vi "listbox_set_values_and_recolor.vi"(4 "item_names":string[][](array[string]), 5 "uneditable_columns":string[](array[string]), 6 "front_panel_reference":refnum<vi>, 7 "column_names":string[](array[string]), 8 "error_in":errorcluster, 9 "Autosize? (T)":bool=TRUE, 10 "Recolor? (T)":bool=TRUE, 11 "multicolumn_listbox_reference_in":refnum<vi>) -> (0 "error_out":errorcluster, 3 "multicolumn_listbox_reference_out":refnum<vi>)   [LabVIEW 2020]
uses:
  <vilib>/Utility/miscctls.llb/LVRowAndColumnTypeDef.ctl
  <vilib>/Utility/miscctls.llb/LVRowAndColumnUnsignedTypeDef.ctl
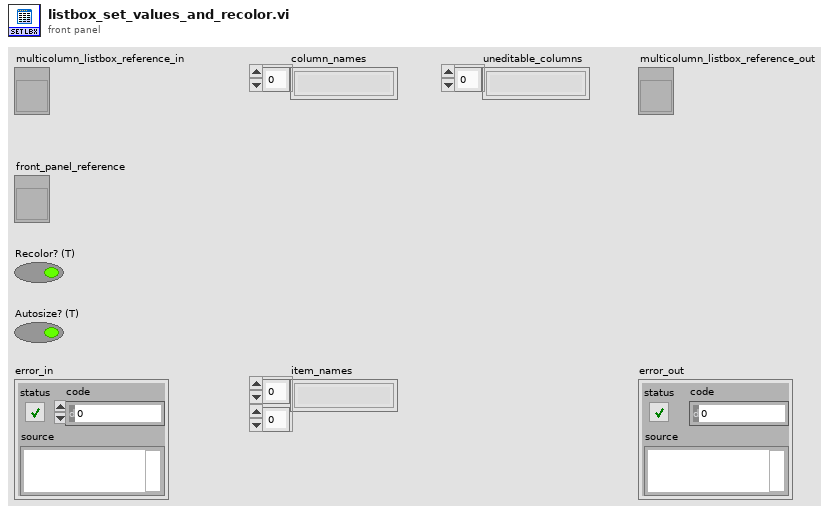
[diagram p1: front panel]
types:
  T1 = typedef "LVRowAndColumnUnsignedTypeDef.ctl" = cluster{"Row":u32, "Column":u32}
  T2 = typedef "LVRowAndColumnTypeDef.ctl" = cluster{"Row":i32, "Column":i32}
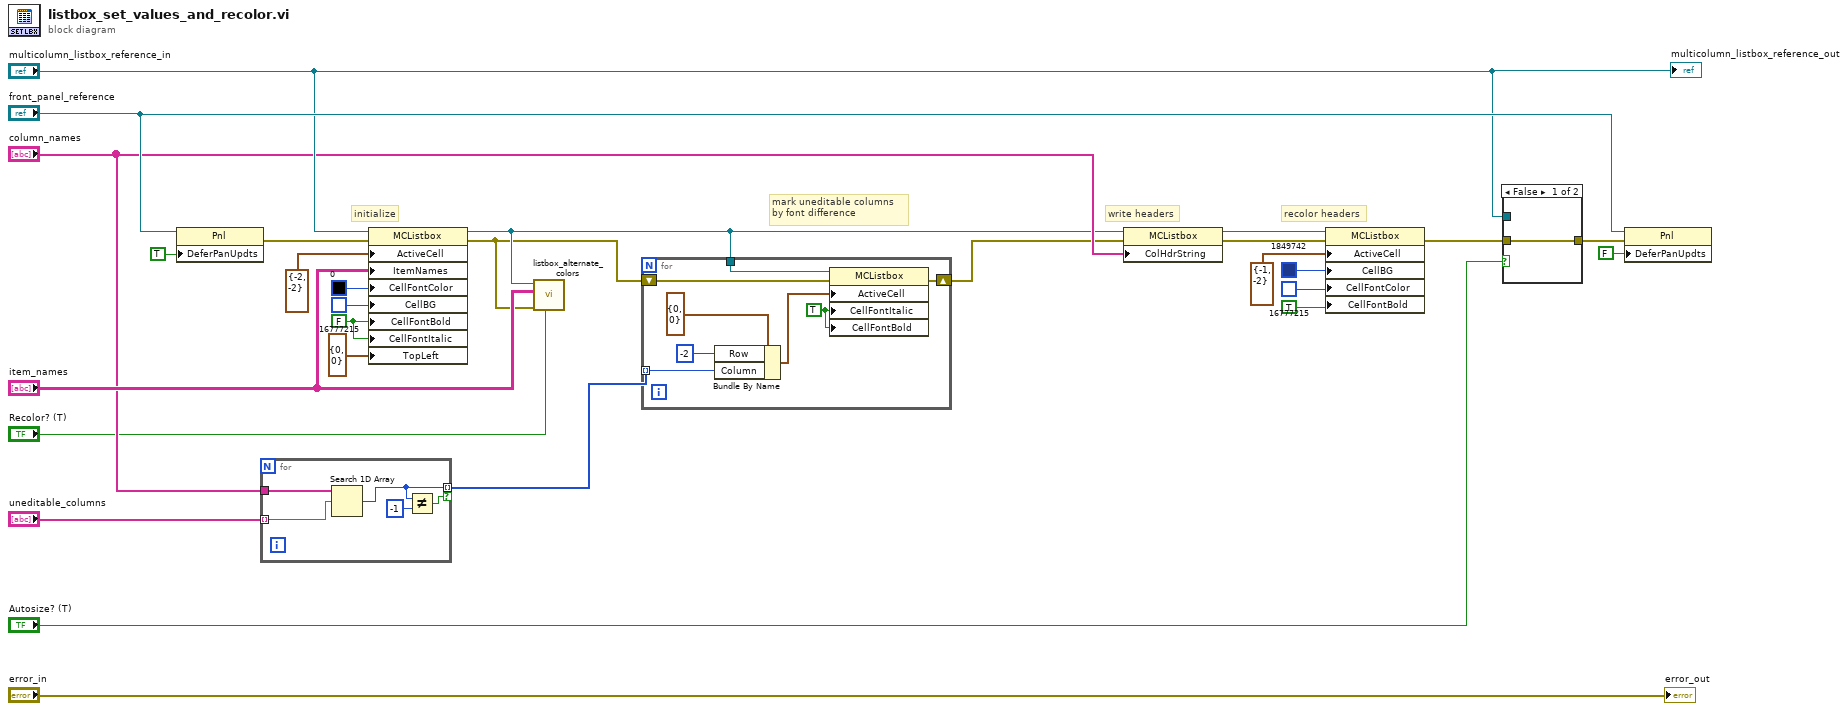
[diagram p0: block diagram]
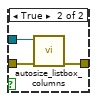
[diagram p2: hidden frame]
diagram:
  w6 = FALSE ("Active Cell:Cell Font:Bold")
  # "mark uneditable columns\nby font difference"
  # "recolor headers"
  # "write headers"
  # "initialize"
  n1 = property on="Property Node" class="Pnl"(reference="front_panel_reference", "DeferPanUpdts"=TRUE ("Defer Panel Updates")) -> (error out=w24:errorcluster)  [unwired: 1 in, 1 out]
  n2 = for {
    tunnel: "column_names" -> [w33]
    tunnel: "uneditable_columns" -> [w32] mode=indexing
    tunnel: [w30] -> w7 mode=indexing if=w31
    n3 = Search 1D Array(1D array=w33, element=w32) -> (index of element=w30:i32)  [unwired: 1 in]
    n4 = Not Equal?(x=w30, y=-1) -> (x != y?=w31:bool)
  }
  n5 = property on="Property Node" class="MCListbox"(reference="multicolumn_listbox_reference_in", error in=w24, "ActiveCell"=T2 {"Row"=-2, "Column"=-2} ("Active Cell:Active Cell"), "ItemNames"="item_names", "CellFontColor"=u32 0, "CellBG"=u32 16777215, "CellFontBold"=w6, "CellFontItalic"=w6, "TopLeft"=T1 {"Row"=0, "Column"=0} ("Top Left Visible Cell")) -> (reference out=w10:refnum<vi>, error out=w9:errorcluster)
  n6 = call "listbox_alternate_colors.vi"("Recolor? (T)"="Recolor? (T)", "error_in"=w9, "item_names"="item_names", "listbox_ref"=w10) -> ()  [unwired: 7 in, 1 out]
  n7 = for {
    tunnel: w10 -> [w41]
    shift-right: [w39] -> w8
    shift-left: w9 -> [w40]
    tunnel: w7 -> [w35] mode=indexing
    w34 = TRUE ("Active Cell:Cell Font:Italic")
    n8 = Bundle By Name(cluster=T2 {"Row"=0, "Column"=0} ("Active Cell:Active Cell"), "Row"=-2, "Column"=w35) -> (w36:T2)
    n9 = property on="Property Node" class="MCListbox"(reference=w41, error in=w40, "ActiveCell"=w36, "CellFontItalic"=w34, "CellFontBold"=w34) -> (error out=w39:errorcluster)  [unwired: 1 out]
  }
  n10 = property on="Property Node" class="MCListbox"(reference=w10, error in=w8, "ColHdrString"="column_names") -> (reference out=w21:refnum<vi>, error out=w20:errorcluster)
  n11 = property on="Property Node" class="MCListbox"(reference=w21, error in=w20, "ActiveCell"=T2 {"Row"=-1, "Column"=-2} ("Active Cell:Active Cell"), "CellBG"=u32 1849742, "CellFontColor"=u32 16777215, "CellFontBold"=TRUE ("Active Cell:Cell Font:Bold")) -> (error out=w15:errorcluster)  [unwired: 1 out]
  n12 = case shown="False" "Autosize? (T)" {
    tunnel: w15 -> [w42 w45]
    tunnel: [w42 w44] -> w14
    tunnel: "multicolumn_listbox_reference_in" -> [_ w43]
    frame False {
    }
    frame True {
      n13 = call "autosize_listbox_columns.vi"("error in (no error)"=w45, "Table Ref"=w43) -> ("error out"=w44:errorcluster)  [unwired: 4 in, 1 out]
    }
  }
  n14 = property on="Property Node" class="Pnl"(reference="front_panel_reference", error in=w14, "DeferPanUpdts"=FALSE ("Defer Panel Updates")) -> ()  [unwired: 2 out]
  "error_out" <- "error_in"
  "multicolumn_listbox_reference_out" <- "multicolumn_listbox_reference_in"
